vi "Tosca-Check DI Connections.vi"(0 "Imaging":T1, 9 "Include required":bool, 11 "error in (no error)":errorcluster) -> (15 "error out":errorcluster)   [LabVIEW 2020]
uses:
  Typedefs/Tosca-Imaging.ctl
  Imaging VIs/Tosca-Imaging Mode.ctl
  Sub VIs/Tosca-Globals.vi
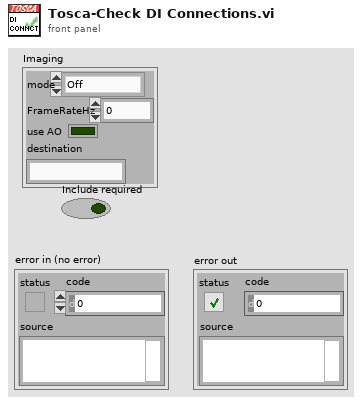
[diagram p1: front panel]
types:
  T1 = typedef "Tosca-Imaging.ctl" = cluster{"mode":T2, "FrameRateHz":dbl, "use AO":bool, "destination":string}
  T2 = typedef "Tosca-Imaging Mode.ctl" = enum16{"Off", "Widefield", "Two-photon"}
  T3 = typedef "CM-Connection.ctl" = cluster{"IOChannel":string, "Endpoint":string}
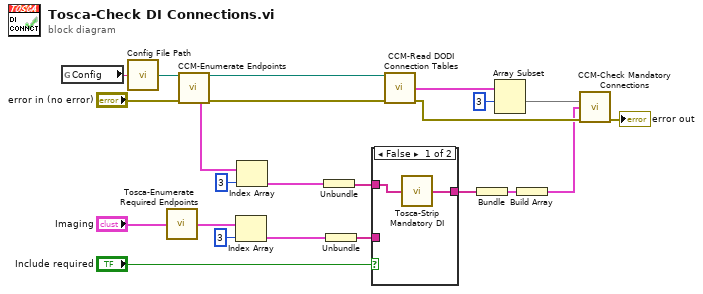
[diagram p0: block diagram]
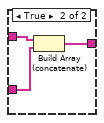
[diagram p2: hidden frame]
diagram:
  n1 = global read "Tosca-Globals.vi" "Config"() -> (w1:string)
  n2 = call "Config File Path.vi"("AppName"=w1) -> ("Default config file name"=w22:path)
  n3 = call "Tosca-Enumerate Required Endpoints.vi"("Imaging"="Imaging") -> ("Required Endpoints"=w16:cluster{string[]}[])  [unwired: 14 in]
  n4 = call "CCM-Enumerate Endpoints.vi"("Path In"=w22, "error in (no error)"="error in (no error)") -> ("Path Out"=w21:path, "Endpoints"=w18:cluster{"Name":string[]}[], "error out"=w20:errorcluster)  [unwired: 9 in, 2 out]
  n5 = Index Array(array=w16, index=3) -> (element=w14:cluster{string[]})
  n6 = Index Array(array=w18, index=3) -> (element=w13:cluster{"Name":string[]})
  n7 = Unbundle(w13) -> ("Name"=w8:string[])
  n8 = Unbundle(w14) -> (w7:string[])
  n9 = case shown="False" "Include required" {
    tunnel: w8 -> [w25 w28]
    tunnel: w7 -> [_ w27]
    tunnel: [w24 w26] -> w6
    frame False {
      n10 = call "Tosca-Strip Mandatory DI.vi"("Digital Signals"=w25) -> ("Filtered DI"=w24:string[])  [unwired: 12 in, 2 out]
    }
    frame True {
      n11 = Build Array (concatenate)(w28, w27) -> (w26:string[])
    }
  }
  n12 = call "CCM-Read DODI Connection Tables.vi"("Path In"=w21, "error in (no error)"=w20) -> ("Tables"=w3:cluster{"Table":T3[]}[], "error out"=w19:errorcluster)  [unwired: 11 in, 1 out]
  n13 = Bundle("Filtered DI"=w6) -> (w11:cluster{"Filtered DI":string[]})  [unwired: 1 in]
  n14 = Array Subset(array=w3, index=3) -> (w4:cluster{"Table":T3[]}[])  [unwired: 1 in]
  n15 = Build Array(w11) -> (w5:cluster{"Filtered DI":string[]}[])
  n16 = call "CCM-Check Mandatory Connections.vi"("Tables"=w4, "Mandatory"=w5, "error in (no error)"=w19) -> ("error out"=→"error out":errorcluster)  [unwired: 11 in, 1 out]
